vi "Global 1.vi"() -> ()   [LabVIEW 2013]
panel:
  in  "Right Encoder Buffer":cluster{"Numeric":dbl, "Numeric 2":dbl}[](array[cluster])
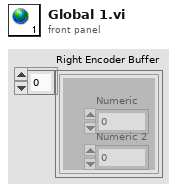
[diagram p1: front panel]
diagram:
